vi "Find Dynamic Test Methods in Test Case.vi"(8 "error in (no error)":errorcluster, 10 "Test Case Class Path":path, 11 "Test Finder In":refnum<class "Test Finder.lvclass">) -> (0 "error out":errorcluster, 2 "Test Methods Out":map{string, path}(c390), 3 "Test Finder Out":refnum<class "Test Finder.lvclass">)   [LabVIEW 2020, in "Test Finder.lvclass"]
uses:
  Test Finder.lvclass
  Test Case/LUnit Test Case.lvclass
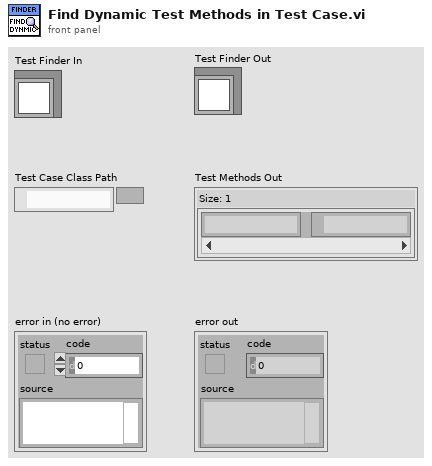
[diagram p1: front panel]
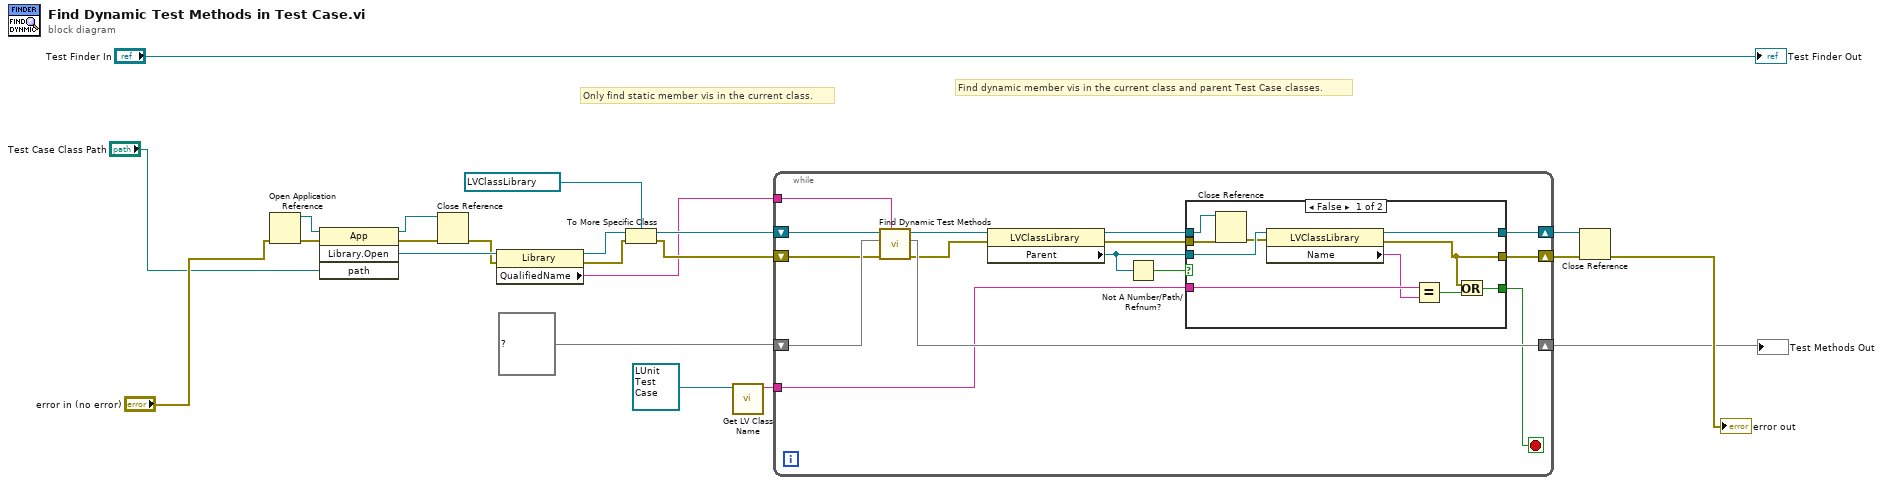
[diagram p0: block diagram]
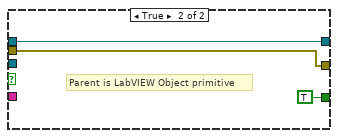
[diagram p2: hidden frame]
diagram:
  # "Find dynamic member vis in the current class and parent Test Case classes."
  # "Only find static member vis in the current class."
  n1 = Open Application Reference(8:"error in (no error)") -> (0:w21:errorcluster, 3:w22:refnum<vi>)  [unwired: 3 in]
  n2 = invoke on="Invoke Node" class="App" method="Library.Open"(reference=w22, error in=w21, "path"="Test Case Class Path") -> (reference out=w19:refnum<vi>, error out=w20:errorcluster, "Open Library"=w7:refnum<vi>)  [unwired: 1 in, 1 out]
  n3 = Close Reference(reference=w19, error in (no error)=w20) -> (error out=w5:errorcluster)
  n4 = property on="Property Node" class="Library"(reference=w7, error in=w5) -> (reference out=w6:refnum<vi>, error out=w4:errorcluster, "QualifiedName"=w2:string)
  n5 = To More Specific Class(target class=refnum<vi> refnum ("Library:Open"), reference=w6, error in=w4) -> (specific class reference=w14:refnum<vi>, error out=w11:errorcluster)
  n6 = call <vilib>:"Get LV Class Name.vi"("object"=refnum<class "LUnit Test Case.lvclass"> refnum ("Test Case in")) -> ("class name"=w13:string)  [unwired: 9 in, 1 out]
  n7 = while {
    shift-right: [w37] -> w8
    shift-left: map{string, path} {} ("Test Methods In") -> [w36]
    shift-right: [w34] -> w15
    shift-left: w14 -> [w33]
    shift-right: [w28] -> w17
    shift-left: w11 -> [w31]
    tunnel: w13 -> [w35]
    tunnel: w2 -> [w23]
    stop <- w29 stop-if-true
    n8 = call "Find Dynamic Test Methods.vi"("Test Case class name"=w23, "error in (no error)"=w31, "Test Methods In"=w36, "LVClassLibrary in"=w33) -> ("error out"=w30:errorcluster, "Test Methods Out"=w37:map{string, path}, "LVClassLibrary out"=w32:refnum<vi>)  [unwired: 5 in]
    n9 = property on="Property Node" class="LVClassLibrary"(reference=w32, error in=w30) -> (reference out=w25:refnum<vi>, error out=w24:errorcluster, "Parent"=w27:refnum<vi>)
    n10 = Not A Number/Path/Refnum?(number/path/refnum=w27) -> (NaN/Path/Refnum?=w26:bool)
    n11 = case shown="False" w26 {
      tunnel: w35 -> [w47 _]
      tunnel: [w46 w49] -> w34
      tunnel: [w45 TRUE] -> w29
      tunnel: [w44 w48] -> w28
      tunnel: w27 -> [w43 _]
      tunnel: w25 -> [w40 w49]
      tunnel: w24 -> [w38 w48]
      frame False {
        n12 = Close Reference(reference=w40, error in (no error)=w38) -> (error out=w39:errorcluster)
        n13 = property on="Property Node" class="LVClassLibrary"(reference=w43, error in=w39) -> (reference out=w46:refnum<vi>, error out=w44:errorcluster, "Name"=w41:string)
        n14 = Equal?(x=w47, y=w41) -> (x = y?=w42:bool)
        n15 = Or(x=w44, y=w42) -> (x .or. y?=w45:bool)
      }
      frame True {
        # "Parent is LabVIEW Object primitive"
      }
    }
  }
  "Test Methods Out" <- w8
  n16 = Close Reference(reference=w15, error in (no error)=w17) -> (error out=→"error out":errorcluster)
  "Test Finder Out" <- "Test Finder In"
